vi "AB_820_850_Project_App_Info.vi"(7 "action":T2, 8 "error in (no error)":errorcluster, 9 "buildType":T1, 10 "applicationInfo in":T3 {"fileType" items=["VFT_UNKNOWN", "VFT_APP", "VFT_DLL", "VFT_DRV", "VFT_FONT", "VFT_VXD", "-", "VFT_STATIC_LIB"]}, 11 "Object In":T4) -> (0 "error out":errorcluster, 2 "Application info":T3 {"fileType" items=["VFT_UNKNOWN", "VFT_APP", "VFT_DLL", "VFT_DRV", "VFT_FONT", "VFT_VXD", "-", "VFT_STATIC_LIB"]}, 3 "Object Out":T4)   [LabVIEW 2020]
uses:
  <resource>/Framework/Providers/API/ItemRef.ctl
  <vilib>/AppBuilder/RW_Project/Compatibility/AB_820_850_Project_App_Data.ctl
  <vilib>/AppBuilder/RW_Project/AB_RW_Project_PropBag_Action.ctl
  <vilib>/AppBuilder/AB_BuildType.ctl
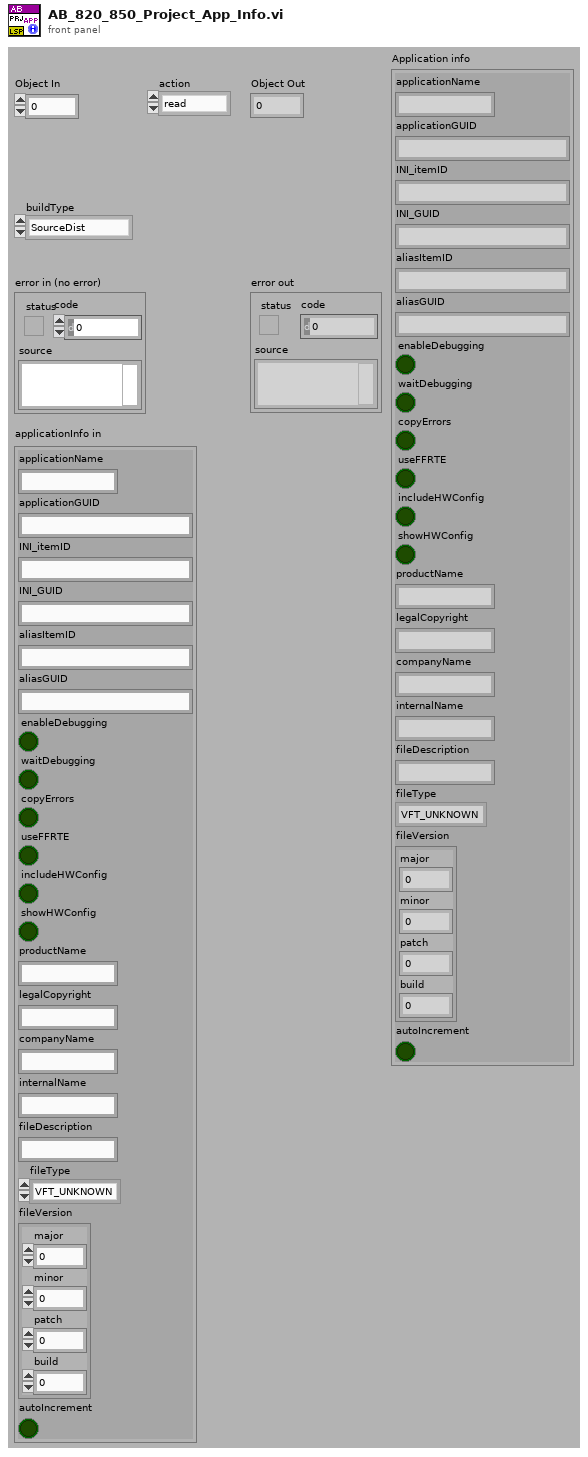
[diagram p1: front panel]
types:
  T1 = typedef "AB_BuildType.ctl" = enum16{"SourceDist", "EXE", "DLL", "RTExe"}
  T2 = typedef "AB_RW_Project_PropBag_Action.ctl" = enum16{"read", "write", "clear", "readPrevious", "writePrevious", "clearPrevious"}
  T3 = typedef "AB_820_850_Project_App_Data.ctl" = cluster{"applicationName":string, "applicationGUID":string, "INI_itemID":string, "INI_GUID":string, "aliasItemID":string, "aliasGUID":string, "enableDebugging":bool, "waitDebugging":bool, "copyErrors":bool, "useFFRTE":bool, "includeHWConfig":bool, "showHWConfig":bool, "productName":string, "legalCopyright":string, "companyName":string, "internalName":string, "fileDescription":string, "fileType":u16, "fileVersion":cluster{"major":u16, "minor":u16, "patch":u16, "build":u16}, "autoIncrement":bool}
  T4 = typedef "ItemRef.ctl" = u64
  T5 = cluster{"[0]":i32, "[1]":i32, "[2]":i32, "[3]":i32}
  T6 = cluster{"major":u16, "minor":u16, "patch":u16, "build":u16}
  T7 = typedef "mxLvPropertyType.ctl" = enum32{"Unknown", "String", "Integer", "Binary", "Reference", "Double", "Unsigned Integer", "Boolean", "XML", "Path"}
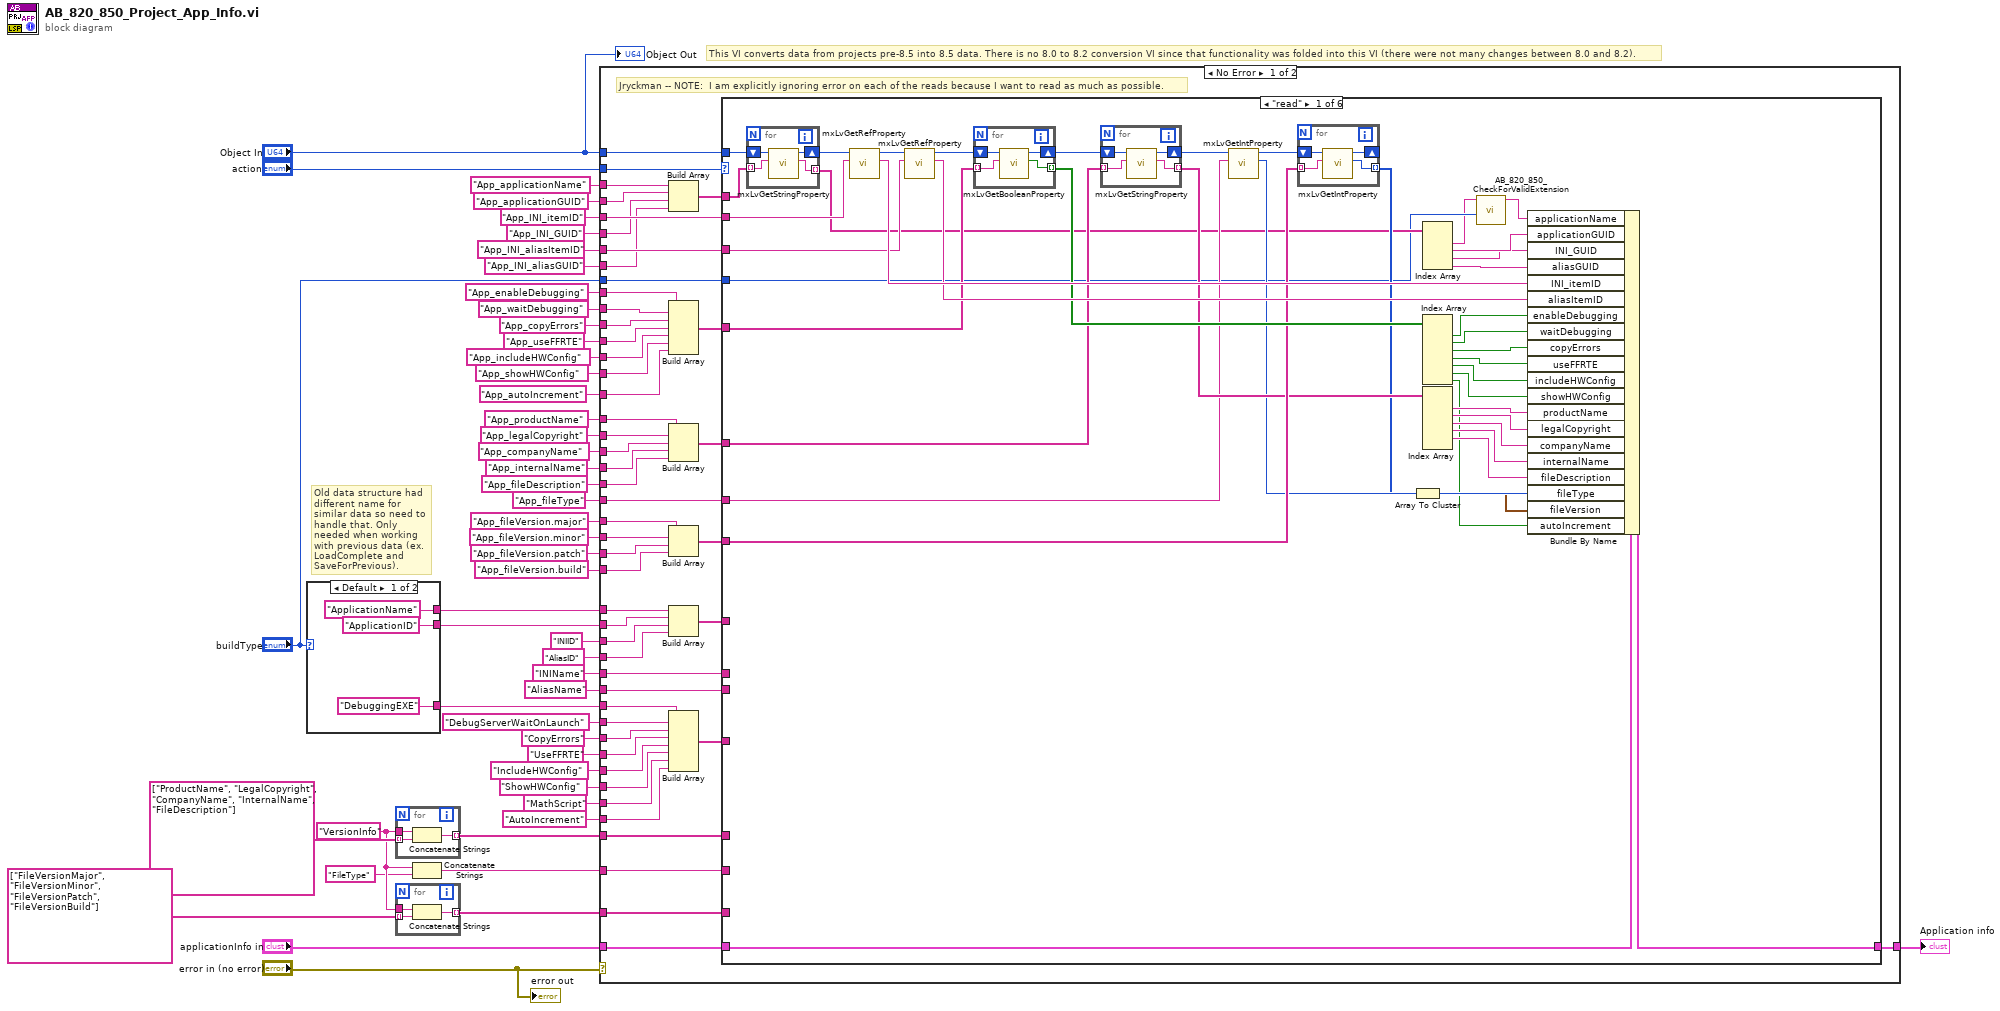
[diagram p0: block diagram]
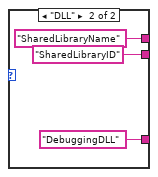
[diagram p2: hidden frame]
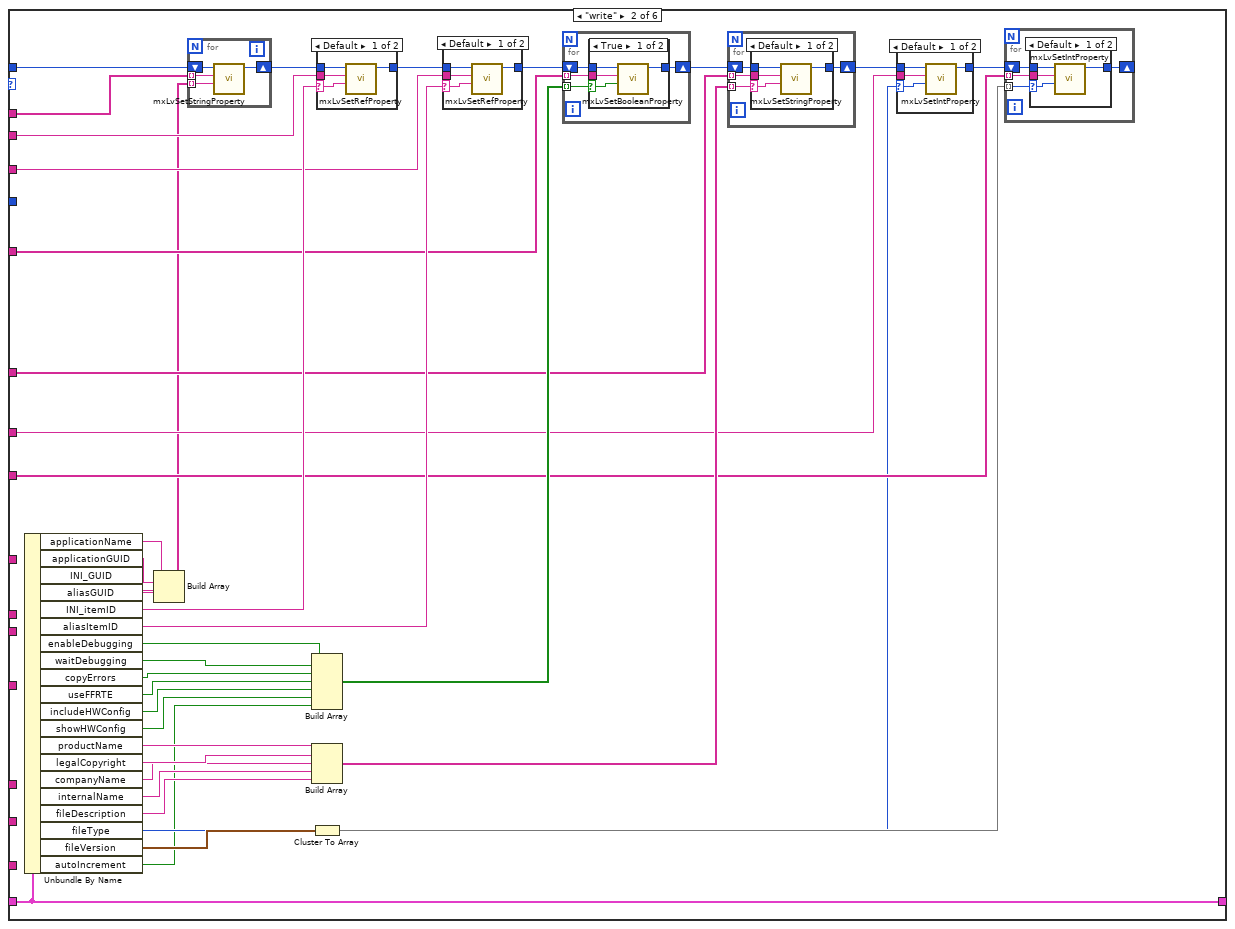
[diagram p3: hidden frame]
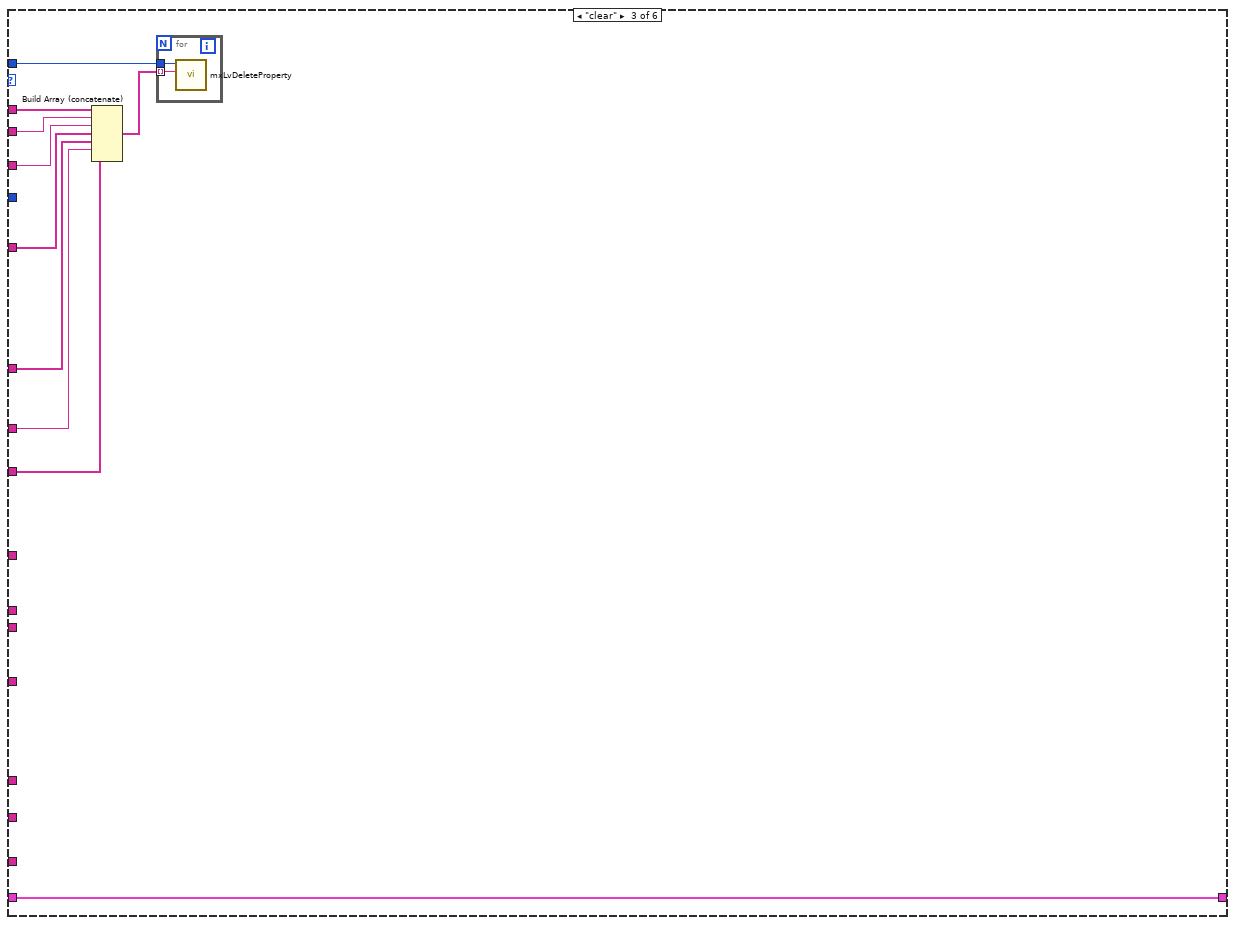
[diagram p10: hidden frame]
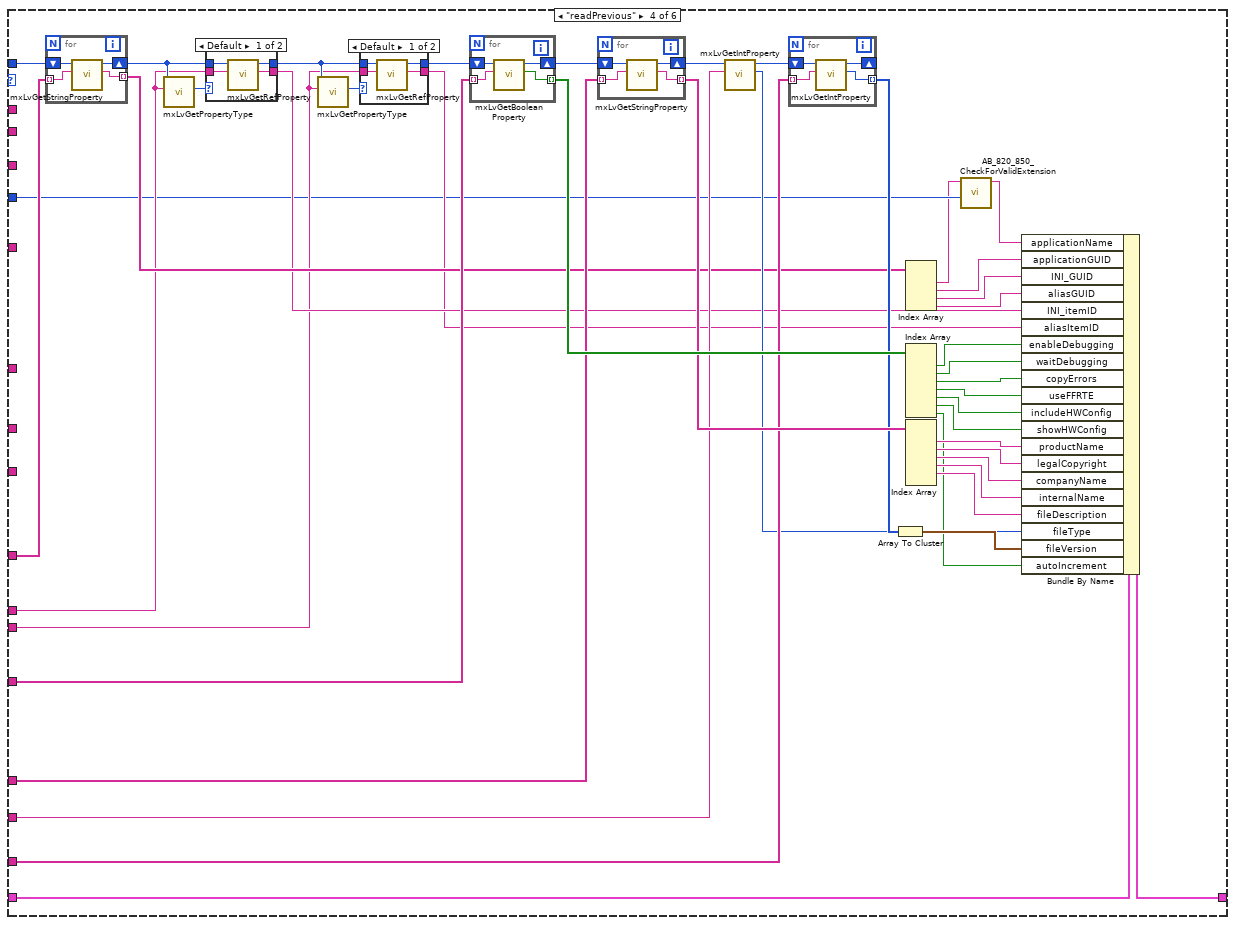
[diagram p11: hidden frame]
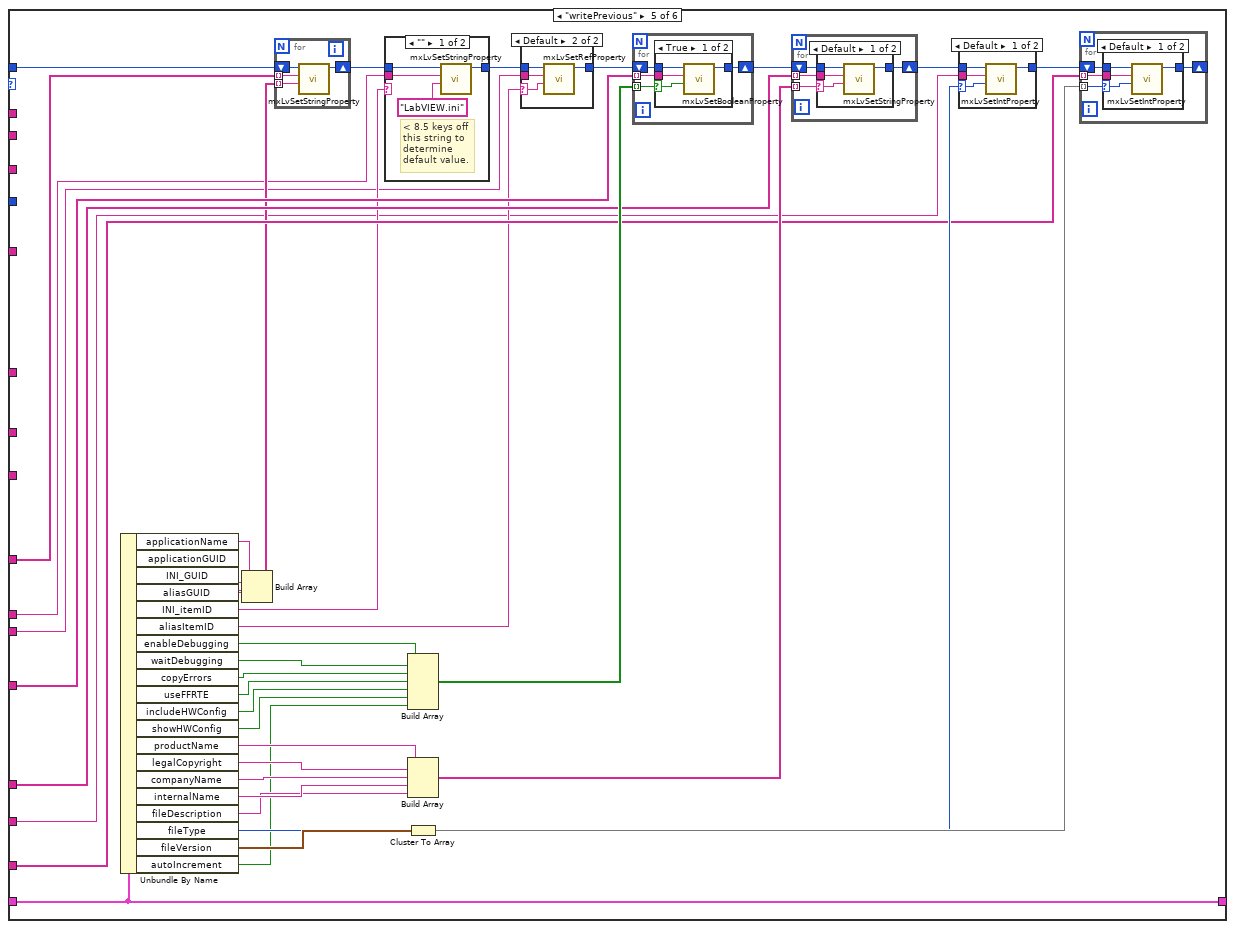
[diagram p14: hidden frame]
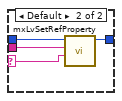
[diagram p16: hidden frame]
diagram:
  w6 = "VersionInfo"
  # "This VI converts data from projects pre-8.5 into 8.5 data. There is no 8.0 to 8.2 conversion VI since that functionality was folded into this VI (there were not many changes between 8.0 and 8.2)."
  # "Old data structure had different name for similar data so need to handle that. Only needed when working with previous data (ex. LoadComplete and SaveForPrevious)."
  n1 = case shown="Default" "buildType" {
    tunnel: ["ApplicationName" "SharedLibraryName"] -> w9
    tunnel: ["ApplicationID" "SharedLibraryID"] -> w8
    tunnel: ["DebuggingEXE" "DebuggingDLL"] -> w7
    frame Default {
    }
    frame "DLL" {
    }
  }
  n2 = for {
    tunnel: w6 -> [w59]
    tunnel: string[] ["ProductName", "LegalCopyright", "CompanyName", "InternalName", "FileDescription"] -> [w58] mode=indexing
    tunnel: [w57] -> w17 mode=indexing
    n3 = Concatenate Strings(w59, w58) -> (w57:string)
  }
  n4 = for {
    tunnel: w6 -> [w62]
    tunnel: string[] ["FileVersionMajor", "FileVersionMinor", "FileVersionPatch", "FileVersionBuild"] -> [w61] mode=indexing
    tunnel: [w60] -> w3 mode=indexing
    n5 = Concatenate Strings(w62, w61) -> (w60:string)
  }
  n6 = Concatenate Strings(w6, "FileType") -> (w2:string)
  n7 = case shown="No Error" "error in (no error)" {
    tunnel: "Object In" -> [w113 _]
    tunnel: [w90 _] -> w48
    tunnel: "applicationInfo in" -> [w96 _]
    tunnel: "App_applicationName" ("Tag") -> [w75 _]
    tunnel: "App_INI_itemID" ("Tag") -> [w112 _]
    tunnel: "App_INI_aliasItemID" ("Tag") -> [w111 _]
    tunnel: "App_enableDebugging" ("Tag") -> [w110 _]
    tunnel: "App_waitDebugging" ("Tag") -> [w109 _]
    tunnel: "App_copyErrors" ("Tag") -> [w108 _]
    tunnel: "App_useFFRTE" ("Tag") -> [w107 _]
    tunnel: "App_includeHWConfig" ("Tag") -> [w106 _]
    tunnel: "App_showHWConfig" ("Tag") -> [w105 _]
    tunnel: "App_productName" ("Tag") -> [w101 _]
    tunnel: "App_legalCopyright" ("Tag") -> [w102 _]
    tunnel: "App_companyName" ("Tag") -> [w100 _]
    tunnel: "App_internalName" ("Tag") -> [w99 _]
    tunnel: "App_fileDescription" ("Tag") -> [w98 _]
    tunnel: "App_fileType" ("Tag") -> [w88 _]
    tunnel: "App_fileVersion.major" ("Tag") -> [w94 _]
    tunnel: "App_fileVersion.minor" ("Tag") -> [w95 _]
    tunnel: "App_fileVersion.patch" ("Tag") -> [w93 _]
    tunnel: "App_fileVersion.build" ("Tag") -> [w92 _]
    tunnel: "App_autoIncrement" ("Tag") -> [w104 _]
    tunnel: "action" -> [w89 _]
    tunnel: w9 -> [w70 _]
    tunnel: "ININame" -> [w87 _]
    tunnel: "AliasName" -> [w86 _]
    tunnel: w7 -> [w85 _]
    tunnel: "DebugServerWaitOnLaunch" -> [w84 _]
    tunnel: "CopyErrors" -> [w79 _]
    tunnel: "UseFFRTE" -> [w83 _]
    tunnel: "IncludeHWConfig" -> [w82 _]
    tunnel: "ShowHWConfig" -> [w81 _]
    tunnel: "MathScript" -> [w80 _]
    tunnel: "AutoIncrement" -> [w78 _]
    tunnel: w17 -> [w77 _]
    tunnel: "App_applicationGUID" ("Tag") -> [w74 _]
    tunnel: "App_INI_GUID" ("Tag") -> [w73 _]
    tunnel: "App_INI_aliasGUID" ("Tag") -> [w72 _]
    tunnel: w8 -> [w69 _]
    tunnel: "INIID" -> [w68 _]
    tunnel: "AliasID" -> [w67 _]
    tunnel: w3 -> [w65 _]
    tunnel: w2 -> [w64 _]
    tunnel: "buildType" -> [w63 _]
    frame No Error {
      # "Jryckman -- NOTE:  I am explicitly ignoring error on each of the reads because I want to read as much as possible."
      n8 = Build Array(w75, w74, w73, w72) -> (w71:string[])
      n9 = Build Array(w110, w109, w108, w107, w106, w105, w104) -> (w103:string[])
      n10 = Build Array(w101, w102, w100, w99, w98) -> (w97:string[])
      n11 = Build Array(w94, w95, w93, w92) -> (w91:string[])
      n12 = Build Array(w70, w69, w68, w67) -> (w66:string[])
      n13 = Build Array(w85, w84, w79, w83, w82, w81, w80, w78) -> (w76:string[])
      n14 = case shown="\"read\"" w89 {
        tunnel: w113 -> [w123 w210 w265 w285 w377 w442]
        tunnel: w112 -> [w151 w208 w264 _ _ _]
        tunnel: w111 -> [w150 w205 w263 _ _ _]
        tunnel: w103 -> [w148 w195 w262 _ _ _]
        tunnel: w97 -> [w138 w193 w261 _ _ _]
        tunnel: w96 -> [w154 w183 w266 w311 w360 w443]
        tunnel: w91 -> [w140 w186 w259 _ _ _]
        tunnel: [w125 w183 w266 w312 w360 w443] -> w90
        tunnel: w88 -> [w129 w179 w260 _ _ _]
        tunnel: w87 -> [_ _ _ w278 w342 w440]
        tunnel: w86 -> [_ _ _ w273 w341 w439]
        tunnel: w77 -> [_ _ _ w300 w355 w437]
        tunnel: w64 -> [_ _ _ w293 w339 w436]
        tunnel: w65 -> [_ _ _ w292 w354 w435]
        tunnel: w76 -> [_ _ _ w288 w356 w438]
        tunnel: w71 -> [w122 w177 w257 _ _ _]
        tunnel: w66 -> [_ _ _ w284 w350 w427]
        tunnel: w63 -> [w116 _ _ w271 _ _]
        frame "read" {
          n15 = for {
            shift-right: [w158] -> w121
            shift-left: w123 -> [w159]
            tunnel: w122 -> [w156] mode=indexing
            tunnel: [w157] -> w120 mode=indexing
            n16 = call <resource>:"mxLvGetStringProperty.vi"("Tag"=w156, "Item"=w159) -> ("Value"=w157:string, "Item"=w158:T4)  [unwired: 7 in, 1 out]
          }
          n17 = call <resource>:"mxLvGetRefProperty.vi"("Tag"=w151, "Item"=w121) -> ("Value"=w153:string, "Item"=w155:T4)  [unwired: 7 in, 1 out]
          n18 = call <resource>:"mxLvGetRefProperty.vi"("Tag"=w150, "Item"=w155) -> ("Value"=w152:string, "Item"=w149:T4)  [unwired: 7 in, 1 out]
          n19 = for {
            shift-right: [w170] -> w139
            shift-left: w149 -> [w171]
            tunnel: w148 -> [w169] mode=indexing
            tunnel: [w168] -> w147 mode=indexing
            n20 = call <resource>:"mxLvGetBooleanProperty.vi"("Tag"=w169, "Item"=w171) -> ("Value"=w168:bool, "Item"=w170:T4)  [unwired: 7 in, 1 out]
          }
          n21 = for {
            shift-right: [w166] -> w131
            shift-left: w139 -> [w167]
            tunnel: w138 -> [w164] mode=indexing
            tunnel: [w165] -> w137 mode=indexing
            n22 = call <resource>:"mxLvGetStringProperty.vi"("Tag"=w164, "Item"=w167) -> ("Value"=w165:string, "Item"=w166:T4)  [unwired: 7 in, 1 out]
          }
          n23 = call <resource>:"mxLvGetIntProperty.vi"("Tag"=w129, "Item"=w131) -> ("Value"=w128:i32, "Item"=w130:T4)  [unwired: 7 in, 1 out]
          n24 = for {
            shift-right: [w162] -> _
            shift-left: w130 -> [w163]
            tunnel: w140 -> [w160] mode=indexing
            tunnel: [w161] -> w127 mode=indexing
            n25 = call <resource>:"mxLvGetIntProperty.vi"("Tag"=w160, "Item"=w163) -> ("Value"=w161:i32, "Item"=w162:T4)  [unwired: 7 in, 1 out]
          }
          n26 = Array To Cluster(array=w127) -> (cluster=w126:T5)
          n27 = Index Array(array=w120) -> (element #1=w115:string, element #2=w119:string, element #3=w118:string, element #4=w117:string)  [unwired: 4 in]
          n28 = Index Array(array=w147) -> (element #1=w146:bool, element #2=w145:bool, element #3=w144:bool, element #4=w143:bool, element #5=w142:bool, element #6=w141:bool, element #7=w124:bool)  [unwired: 7 in]
          n29 = Index Array(array=w137) -> (element #1=w136:string, element #2=w135:string, element #3=w134:string, element #4=w133:string, element #5=w132:string)  [unwired: 6 in, 1 out]
          n30 = call <vilib>:"AB_820_850_CheckForValidExtension.vi"("buildType"=w116, "Filename in"=w115) -> ("Filename out"=w114:string)  [unwired: 8 in, 1 out]
          n31 = Bundle By Name(cluster=w154, "applicationName"=w114, "applicationGUID"=w119, "INI_GUID"=w118, "aliasGUID"=w117, "INI_itemID"=w153, "aliasItemID"=w152, "enableDebugging"=w146, "waitDebugging"=w145, "copyErrors"=w144, "useFFRTE"=w143, "includeHWConfig"=w142, "showHWConfig"=w141, "productName"=w136, "legalCopyright"=w135, "companyName"=w134, "internalName"=w133, "fileDescription"=w132, "fileType"=w128, "fileVersion"=w126, "autoIncrement"=w124) -> (w125:T3)
        }
        frame "write" {
          n32 = Unbundle By Name(w183) -> ("applicationName"=w176:string, "applicationGUID"=w175:string, "INI_GUID"=w172:string, "aliasGUID"=w174:string, "INI_itemID"=w207:string, "aliasItemID"=w204:string, "enableDebugging"=w197:bool, "waitDebugging"=w202:bool, "copyErrors"=w201:bool, "useFFRTE"=w200:bool, "includeHWConfig"=w199:bool, "showHWConfig"=w198:bool, "productName"=w191:string, "legalCopyright"=w192:string, "companyName"=w190:string, "internalName"=w189:string, "fileDescription"=w188:string, "fileType"=w180:u16, "fileVersion"=w185:T6, "autoIncrement"=w178:bool)
          n33 = Build Array(w176, w175, w172, w174) -> (w173:string[])
          n34 = for {
            tunnel: w177 -> [w212] mode=indexing
            tunnel: w173 -> [w211] mode=indexing
            shift-right: [w213] -> w209
            shift-left: w210 -> [w214]
            n35 = call <resource>:"mxLvSetStringProperty.vi"("Value (\"\")"=w211, "Tag"=w212, "Item"=w214) -> ("Item"=w213:T4)  [unwired: 7 in, 1 out]
          }
          n36 = Build Array(w197, w202, w201, w200, w199, w198, w178) -> (w196:bool[])
          n37 = Build Array(w191, w192, w190, w189, w188) -> (w187:string[])
          n38 = Cluster To Array(cluster=w185) -> (array=w184:u16[])
          n39 = case shown="Default" w207 {
            selector: w207 -> [w253 _]
            tunnel: w209 -> [w255 w256]
            tunnel: w208 -> [w254 _]
            tunnel: [w252 w256] -> w206
            frame Default {
              n40 = call <resource>:"mxLvSetRefProperty.vi"("Value (\"\")"=w253, "Tag"=w254, "Item"=w255) -> ("Item"=w252:T4)  [unwired: 7 in, 1 out]
            }
            frame "" {
            }
          }
          n41 = case shown="Default" w204 {
            selector: w204 -> [w248 _]
            tunnel: w206 -> [w250 w251]
            tunnel: w205 -> [w249 _]
            tunnel: [w247 w251] -> w203
            frame Default {
              n42 = call <resource>:"mxLvSetRefProperty.vi"("Value (\"\")"=w248, "Tag"=w249, "Item"=w250) -> ("Item"=w247:T4)  [unwired: 7 in, 1 out]
            }
            frame "" {
            }
          }
          n43 = for {
            tunnel: w196 -> [w240] mode=indexing
            shift-right: [w239] -> w194
            shift-left: w203 -> [w241]
            tunnel: w195 -> [w238] mode=indexing
            n44 = case shown="True" w240 {
              selector: w240 -> [w244 _]
              tunnel: w241 -> [w245 w246]
              tunnel: w238 -> [w242 _]
              tunnel: [w243 w246] -> w239
              frame True {
                n45 = call <resource>:"mxLvSetBooleanProperty.vi"("Value (F)"=w244, "Tag"=w242, "Item"=w245) -> ("Item"=w243:T4)  [unwired: 7 in, 1 out]
              }
              frame False {
              }
            }
          }
          n46 = for {
            tunnel: w187 -> [w231] mode=indexing
            shift-right: [w230] -> w182
            shift-left: w194 -> [w232]
            tunnel: w193 -> [w229] mode=indexing
            n47 = case shown="Default" w231 {
              selector: w231 -> [w234 _]
              tunnel: w232 -> [w236 w237]
              tunnel: w229 -> [w233 _]
              tunnel: [w235 w237] -> w230
              frame Default {
                n48 = call <resource>:"mxLvSetStringProperty.vi"("Value (\"\")"=w234, "Tag"=w233, "Item"=w236) -> ("Item"=w235:T4)  [unwired: 7 in, 1 out]
              }
              frame "" {
              }
            }
          }
          n49 = case shown="Default" w180 {
            selector: w180 -> [w217 _]
            tunnel: w182 -> [w218 w219]
            tunnel: w179 -> [w216 _]
            tunnel: [w215 w219] -> w181
            frame Default {
              n50 = call <resource>:"mxLvSetIntProperty.vi"("Value (0)"=w217, "Tag"=w216, "Item"=w218) -> ("Item"=w215:T4)  [unwired: 7 in, 1 out]
            }
            frame 0 {
            }
          }
          n51 = for {
            tunnel: w184 -> [w222] mode=indexing
            shift-right: [w221] -> _
            shift-left: w181 -> [w223]
            tunnel: w186 -> [w220] mode=indexing
            n52 = case shown="Default" w222 {
              selector: w222 -> [w226 _]
              tunnel: w223 -> [w227 w228]
              tunnel: w220 -> [w225 _]
              tunnel: [w224 w228] -> w221
              frame Default {
                n53 = call <resource>:"mxLvSetIntProperty.vi"("Value (0)"=w226, "Tag"=w225, "Item"=w227) -> ("Item"=w224:T4)  [unwired: 7 in, 1 out]
              }
              frame 0 {
              }
            }
          }
        }
        frame "clear" {
          n54 = Build Array (concatenate)(w257, w264, w263, w262, w261, w260, w259) -> (w258:string[])
          n55 = for {
            tunnel: w265 -> [w268]
            tunnel: w258 -> [w267] mode=indexing
            n56 = call <resource>:"mxLvDeleteProperty.vi"("Tag"=w267, "Item"=w268) -> ()  [unwired: 8 in, 2 out]
          }
        }
        frame "readPrevious" {
          n57 = for {
            shift-right: [w320] -> w279
            shift-left: w285 -> [w321]
            tunnel: w284 -> [w318] mode=indexing
            tunnel: [w319] -> w283 mode=indexing
            n58 = call <resource>:"mxLvGetStringProperty.vi"("Tag"=w318, "Item"=w321) -> ("Value"=w319:string, "Item"=w320:T4)  [unwired: 7 in, 1 out]
          }
          n59 = call <resource>:"mxLvGetPropertyType.vi"("Tag"=w278, "Item"=w279) -> ("Type"=w286:T7)  [unwired: 7 in, 2 out]
          n60 = case shown="Default" w286 {
            tunnel: w279 -> [w325 w326]
            tunnel: w278 -> [w323 _]
            tunnel: [w324 _] -> w277
            tunnel: [w322 w326] -> w275
            frame Default {
              n61 = call <resource>:"mxLvGetRefProperty.vi"("Tag"=w323, "Item"=w325) -> ("Value"=w324:string, "Item"=w322:T4)  [unwired: 7 in, 1 out]
            }
            frame "String" {
            }
          }
          n62 = call <resource>:"mxLvGetPropertyType.vi"("Tag"=w273, "Item"=w275) -> ("Type"=w276:T7)  [unwired: 7 in, 2 out]
          n63 = case shown="Default" w276 {
            tunnel: w275 -> [w316 w317]
            tunnel: w273 -> [w314 _]
            tunnel: [w315 _] -> w272
            tunnel: [w313 w317] -> w274
            frame Default {
              n64 = call <resource>:"mxLvGetRefProperty.vi"("Tag"=w314, "Item"=w316) -> ("Value"=w315:string, "Item"=w313:T4)  [unwired: 7 in, 1 out]
            }
            frame "String" {
            }
          }
          n65 = for {
            shift-right: [w337] -> w301
            shift-left: w274 -> [w338]
            tunnel: [w336] -> w309 mode=indexing
            tunnel: w288 -> [w335] mode=indexing
            n66 = call <resource>:"mxLvGetBooleanProperty.vi"("Tag"=w335, "Item"=w338) -> ("Value"=w336:bool, "Item"=w337:T4)  [unwired: 7 in, 1 out]
          }
          n67 = for {
            shift-right: [w333] -> w303
            shift-left: w301 -> [w334]
            tunnel: w300 -> [w331] mode=indexing
            tunnel: [w332] -> w299 mode=indexing
            n68 = call <resource>:"mxLvGetStringProperty.vi"("Tag"=w331, "Item"=w334) -> ("Value"=w332:string, "Item"=w333:T4)  [unwired: 7 in, 1 out]
          }
          n69 = call <resource>:"mxLvGetIntProperty.vi"("Tag"=w293, "Item"=w303) -> ("Value"=w289:i32, "Item"=w302:T4)  [unwired: 7 in, 1 out]
          n70 = for {
            shift-right: [w329] -> _
            shift-left: w302 -> [w330]
            tunnel: w292 -> [w327] mode=indexing
            tunnel: [w328] -> w291 mode=indexing
            n71 = call <resource>:"mxLvGetIntProperty.vi"("Tag"=w327, "Item"=w330) -> ("Value"=w328:i32, "Item"=w329:T4)  [unwired: 7 in, 1 out]
          }
          n72 = Array To Cluster(array=w291) -> (cluster=w290:T5)
          n73 = Index Array(array=w283) -> (element #1=w270:string, element #2=w282:string, element #3=w281:string, element #4=w280:string)  [unwired: 4 in]
          n74 = Index Array(array=w309) -> (element #1=w310:bool, element #2=w308:bool, element #3=w307:bool, element #4=w306:bool, element #5=w305:bool, element #6=w304:bool, element #7=w287:bool)  [unwired: 7 in]
          n75 = Index Array(array=w299) -> (element #1=w298:string, element #2=w297:string, element #3=w296:string, element #4=w295:string, element #5=w294:string)  [unwired: 6 in, 1 out]
          n76 = call <vilib>:"AB_820_850_CheckForValidExtension.vi"("buildType"=w271, "Filename in"=w270) -> ("Filename out"=w269:string)  [unwired: 8 in, 1 out]
          n77 = Bundle By Name(cluster=w311, "applicationName"=w269, "applicationGUID"=w282, "INI_GUID"=w281, "aliasGUID"=w280, "INI_itemID"=w277, "aliasItemID"=w272, "enableDebugging"=w310, "waitDebugging"=w308, "copyErrors"=w307, "useFFRTE"=w306, "includeHWConfig"=w305, "showHWConfig"=w304, "productName"=w298, "legalCopyright"=w297, "companyName"=w296, "internalName"=w295, "fileDescription"=w294, "fileType"=w289, "fileVersion"=w290, "autoIncrement"=w287) -> (w312:T3)
        }
        frame "writePrevious" {
          n78 = Unbundle By Name(w360) -> ("applicationName"=w347:string, "applicationGUID"=w348:string, "INI_GUID"=w349:string, "aliasGUID"=w346:string, "INI_itemID"=w352:string, "aliasItemID"=w340:string, "enableDebugging"=w371:bool, "waitDebugging"=w376:bool, "copyErrors"=w375:bool, "useFFRTE"=w374:bool, "includeHWConfig"=w373:bool, "showHWConfig"=w372:bool, "productName"=w367:string, "legalCopyright"=w368:string, "companyName"=w366:string, "internalName"=w365:string, "fileDescription"=w364:string, "fileType"=w357:u16, "fileVersion"=w362:T6, "autoIncrement"=w353:bool)
          n79 = Build Array(w347, w348, w349, w346) -> (w345:string[])
          n80 = for {
            tunnel: w345 -> [w380] mode=indexing
            tunnel: w350 -> [w379] mode=indexing
            shift-right: [w378] -> w344
            shift-left: w377 -> [w381]
            n81 = call <resource>:"mxLvSetStringProperty.vi"("Value (\"\")"=w380, "Tag"=w379, "Item"=w381) -> ("Item"=w378:T4)  [unwired: 7 in, 1 out]
          }
          n82 = case shown="\"\"" w352 {
            selector: w352 -> [_ w391]
            tunnel: w344 -> [w390 w394]
            tunnel: w342 -> [w388 w393]
            tunnel: [w389 w392] -> w351
            frame "" {
              # "< 8.5 keys off this string to determine default value."
              n83 = call <resource>:"mxLvSetStringProperty.vi"("Value (\"\")"="LabVIEW.ini", "Tag"=w388, "Item"=w390) -> ("Item"=w389:T4)  [unwired: 7 in, 1 out]
            }
            frame Default {
              n84 = call <resource>:"mxLvSetRefProperty.vi"("Value (\"\")"=w391, "Tag"=w393, "Item"=w394) -> ("Item"=w392:T4)  [unwired: 7 in, 1 out]
            }
          }
          n85 = Build Array(w371, w376, w375, w374, w373, w372, w353) -> (w370:bool[])
          n86 = Build Array(w367, w368, w366, w365, w364) -> (w363:string[])
          n87 = Cluster To Array(cluster=w362) -> (array=w361:u16[])
          n88 = case shown="Default" w340 {
            selector: w340 -> [_ w383]
            tunnel: w351 -> [w382 w386]
            tunnel: w341 -> [_ w385]
            tunnel: [w382 w384] -> w343
            frame "" {
            }
            frame Default {
              n89 = call <resource>:"mxLvSetRefProperty.vi"("Value (\"\")"=w383, "Tag"=w385, "Item"=w386) -> ("Item"=w384:T4)  [unwired: 7 in, 1 out]
            }
          }
          n90 = for {
            tunnel: w370 -> [w420] mode=indexing
            shift-right: [w419] -> w369
            shift-left: w343 -> [w421]
            tunnel: w356 -> [w418] mode=indexing
            n91 = case shown="True" w420 {
              selector: w420 -> [w424 _]
              tunnel: w421 -> [w425 w426]
              tunnel: w418 -> [w422 _]
              tunnel: [w423 w426] -> w419
              frame True {
                n92 = call <resource>:"mxLvSetBooleanProperty.vi"("Value (F)"=w424, "Tag"=w422, "Item"=w425) -> ("Item"=w423:T4)  [unwired: 7 in, 1 out]
              }
              frame False {
              }
            }
          }
          n93 = for {
            tunnel: w363 -> [w411] mode=indexing
            shift-right: [w410] -> w359
            shift-left: w369 -> [w412]
            tunnel: w355 -> [w409] mode=indexing
            n94 = case shown="Default" w411 {
              selector: w411 -> [w414 _]
              tunnel: w412 -> [w416 w417]
              tunnel: w409 -> [w413 _]
              tunnel: [w415 w417] -> w410
              frame Default {
                n95 = call <resource>:"mxLvSetStringProperty.vi"("Value (\"\")"=w414, "Tag"=w413, "Item"=w416) -> ("Item"=w415:T4)  [unwired: 7 in, 1 out]
              }
              frame "" {
              }
            }
          }
          n96 = case shown="Default" w357 {
            selector: w357 -> [w397 _]
            tunnel: w359 -> [w398 w399]
            tunnel: w339 -> [w396 _]
            tunnel: [w395 w399] -> w358
            frame Default {
              n97 = call <resource>:"mxLvSetIntProperty.vi"("Value (0)"=w397, "Tag"=w396, "Item"=w398) -> ("Item"=w395:T4)  [unwired: 7 in, 1 out]
            }
            frame 0 {
            }
          }
          n98 = for {
            tunnel: w361 -> [w402] mode=indexing
            shift-right: [w401] -> _
            shift-left: w358 -> [w403]
            tunnel: w354 -> [w400] mode=indexing
            n99 = case shown="Default" w402 {
              selector: w402 -> [w406 _]
              tunnel: w403 -> [w407 w408]
              tunnel: w400 -> [w405 _]
              tunnel: [w404 w408] -> w401
              frame Default {
                n100 = call <resource>:"mxLvSetIntProperty.vi"("Value (0)"=w406, "Tag"=w405, "Item"=w407) -> ("Item"=w404:T4)  [unwired: 7 in, 1 out]
              }
              frame 0 {
              }
            }
          }
        }
        frame "clearPrevious" {
          # "Legacy tokens"
          n101 = Build Array("ININame", "AliasName", "ApplicationID", "TLBID", "LOGID", "IncludeSCC" ("Tag")) -> (w428:string[])
          n102 = Build Array (concatenate)(w427, w440, w439, w438, w437, w436, w435, w428) -> (w441:string[])
          n103 = for {
            tunnel: w442 -> [w445]
            tunnel: w441 -> [w444] mode=indexing
            n104 = call <resource>:"mxLvDeleteProperty.vi"("Tag"=w444, "Item"=w445) -> ()  [unwired: 8 in, 2 out]
          }
        }
      }
    }
    frame Error {
    }
  }
  "Application info" <- w48
  "Object Out" <- "Object In"
  "error out" <- "error in (no error)"
